vi "TriggerThresholdCrossed.vi"(8 "Threshold":dbl format="%0.2f", 9 "Last":dbl format="%0.2f", 10 "Current":dbl format="%0.2f", 11 "Sense":T1) -> (2 "Satisfied":bool)   [LabVIEW 2013]
uses:
  <vilib>/express/express signal manip/TriggerBlock.llb/triggerSense.ctl
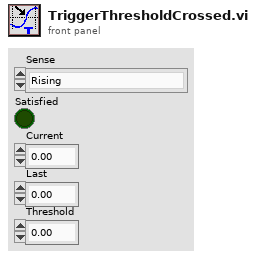
[diagram p1: front panel]
types:
  T1 = typedef "triggerSense.ctl" = enum32{"Rising", "Rising or Falling", "Falling"}
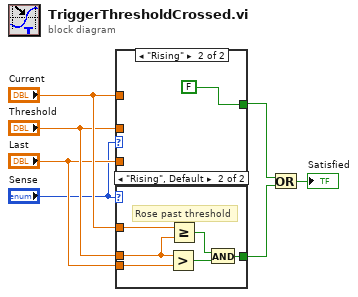
[diagram p0: block diagram]
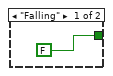
[diagram p2: hidden frame]
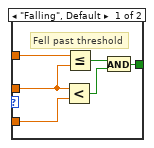
[diagram p3: hidden frame]
diagram:
  n1 = case shown="\"Rising\"" "Sense" {
    tunnel: "Current" -> [w13 _]
    tunnel: "Last" -> [w12 _]
    tunnel: "Threshold" -> [w11 _]
    tunnel: [w8 FALSE] -> w3
    frame "Falling", Default {
      # "Fell past threshold"
      n2 = Less?(x=w11, y=w12) -> (x < y?=w9:bool)
      n3 = Less Or Equal?(x=w13, y=w11) -> (x <= y?=w10:bool)
      n4 = And(x=w10, y=w9) -> (x .and. y?=w8:bool)
    }
    frame "Rising" {
    }
  }
  n5 = case shown="\"Rising\", Default" "Sense" {
    tunnel: "Current" -> [_ w21]
    tunnel: "Last" -> [_ w20]
    tunnel: "Threshold" -> [_ w19]
    tunnel: [FALSE w18] -> w2
    frame "Falling" {
    }
    frame "Rising", Default {
      # "Rose past threshold"
      n6 = Greater?(x=w19, y=w20) -> (0:w17:bool)
      n7 = Greater Or Equal?(x=w21, y=w19) -> (x >= y?=w16:bool)
      n8 = And(x=w16, y=w17) -> (x .and. y?=w18:bool)
    }
  }
  n9 = Or(x=w3, y=w2) -> (x .or. y?=→"Satisfied":bool)
